vi "SimpleLink.vi"(0 "Geometry":string, 1 "Name":string, 2 "origin":T1, 3 "mass":dbl=1.0, 4 "link color":u32(colorbox)=16712704) -> (5 "link out":string)   [LabVIEW 2012]
uses:
  <vilib>/Analysis/Matrix/Datatypes/RealMatrix.ctl
  <userlib>/rosforlv/Gazebo/URDF_conversion/CollisionAttributes.ctl
  <userlib>/rosforlv/Gazebo/URDF_conversion/VisionAttributes.ctl
  <userlib>/rosforlv/Gazebo/URDF_conversion/InertiaAttributes.ctl
  <userlib>/rosforlv/Gazebo/URDF_conversion/LinkAttributes.ctl
  <vilib>/Analysis/Matrix/NI_Matrix.lvlib
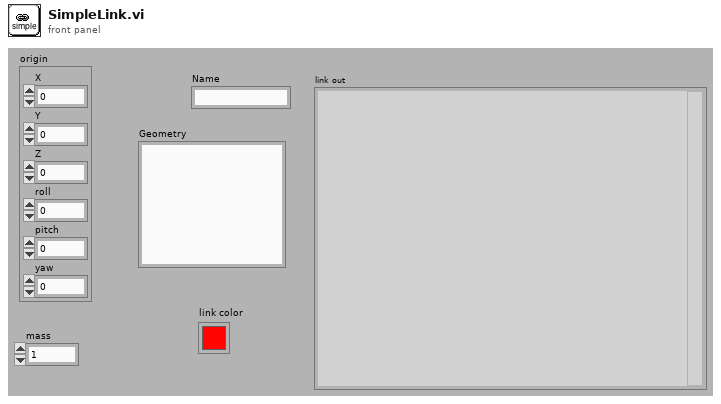
[diagram p1: front panel]
types:
  T1 = cluster{"X":sgl, "Y":sgl, "Z":sgl, "roll":sgl, "pitch":sgl, "yaw":sgl}
  T2 = typedef "LinkAttributes.ctl" = cluster{"inertia":string, "visual":string, "collision":string}
  T3 = typedef "InertiaAttributes.ctl" = cluster{"origin":string, "mass":string}
  T4 = typedef "VisionAttributes.ctl" = cluster{"name":string, "origin":string, "geometry":string, "material":string}
  T5 = typedef "CollisionAttributes.ctl" = cluster{"name":string, "origin":string, "geometry":string}
  T6 = typedef "NI_Matrix.lvlib/RealMatrix.ctl" = dbl[][]
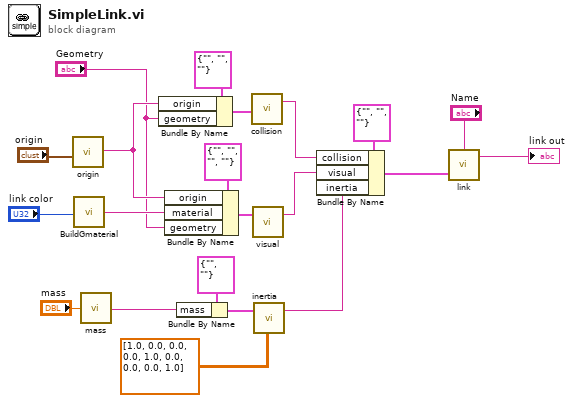
[diagram p0: block diagram]
diagram:
  n1 = call <userlib>:"origin.vi"("origin"="origin") -> ("urdf out"=w13:string)
  n2 = call <userlib>:"BuildGmaterial.vi"("link color"="link color") -> ("sdf"=w14:string)  [unwired: 1 in]
  n3 = call <userlib>:"mass.vi"("mass"="mass") -> ("urdf"=w8:string)
  n4 = Bundle By Name(cluster=T5 {"name"="", "origin"="", "geometry"=""} ("Attributes"), "origin"=w13, "geometry"="Geometry") -> (w12:T5)
  n5 = Bundle By Name(cluster=T4 {"name"="", "origin"="", "geometry"="", "material"=""} ("Attributes"), "origin"=w13, "material"=w14, "geometry"="Geometry") -> (w17:T4)
  n6 = Bundle By Name(cluster=T3 {"origin"="", "mass"=""} ("Attributes"), "mass"=w8) -> (w9:T3)
  n7 = call <userlib>:"collision.vi"("Attributes"=w12) -> ("urdf out"=w21:string)  [unwired: 3 in]
  n8 = call <userlib>:"visual.vi"("Attributes"=w17) -> ("urdf out"=w20:string)  [unwired: 3 in]
  n9 = call <userlib>:"inertia.vi"("Inertia"=T6 [[1.0, 0.0, 0.0], [0.0, 1.0, 0.0], [0.0, 0.0, 1.0]], "Attributes"=w9) -> ("sdf out"=w11:string)  [unwired: 2 in]
  n10 = Bundle By Name(cluster=T2 {"inertia"="", "visual"="", "collision"=""} ("Attributes"), "collision"=w21, "visual"=w20, "inertia"=w11) -> (w6:T2)
  n11 = call <userlib>:"link.vi"("Attributes"=w6, "Name"="Name") -> ("urdf out"=→"link out":string)  [unwired: 2 in]
